vi "SE_HV500.contents.vi"   [LabVIEW 2014, in "SE_HV500.lvlib"]
uses:
  SE_HV500.lvlib
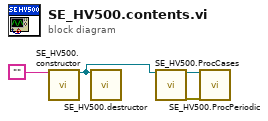
[diagram p0: block diagram]
diagram:
  n1 = call "SE_HV500.constructor.vi"("name"="") -> ("i ref out"=w1:refnum<vi>)  [unwired: 16 in, 2 out]
  n2 = call "SE_HV500.destructor.vi"("i ref in"=w1) -> ()  [unwired: 18 in, 1 out]
  n3 = call "SE_HV500.ProcCases.vi"("i ref in"=w1) -> ("i ref out"=w4:refnum<vi>, "error out"=w3:errorcluster)  [unwired: 16 in, 1 out]
  n4 = call "SE_HV500.ProcPeriodic.vi"("i ref in"=w4, "error in (no error)"=w3) -> ()  [unwired: 15 in, 3 out]
